vi "Get Hardware Version.vi"(0 "PCB":u32, 1 "Decode":u32, 2 "dummy1":u32, 3 "dummy2":u32, 4 "CameraFirmwareVersion":u32, 5 "CameraFirmwareBuild":u32, 7 "error in (no error)":errorcluster) -> (20 "PCB out":u32, 21 "Decode out":u32, 22 "dummy1 out":u32, 23 "dummy2 out":u32, 24 "CameraFirmwareVersion out":u32, 25 "CameraFirmwareBuild out":u32, 26 "function return":u32, 27 "error out":errorcluster)   [LabVIEW 2014, in "atmcd32d.lvlib"]
doc: "unsigned int WINAPI GetHardwareVersion(unsigned int * PCB, unsigned int * Decode, unsigned int * dummy1, unsigned int * dummy2, unsigned int * CameraFirmwareVersion, unsigned int * CameraFirmwareBuild);"
uses:
  atmcd32d.lvlib
  atmcd32d.dll
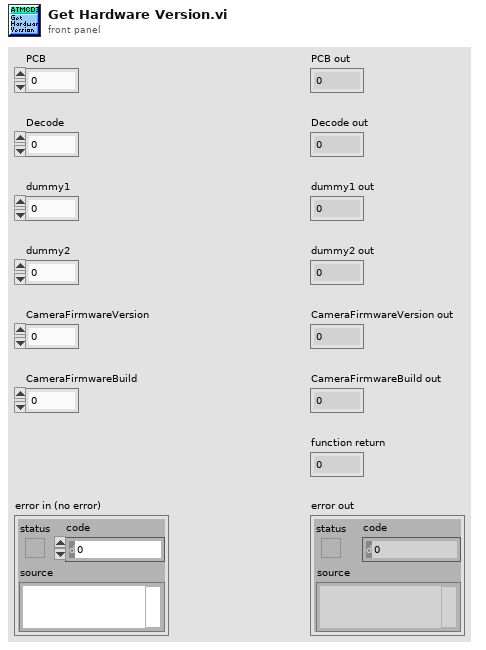
[diagram p1: front panel]
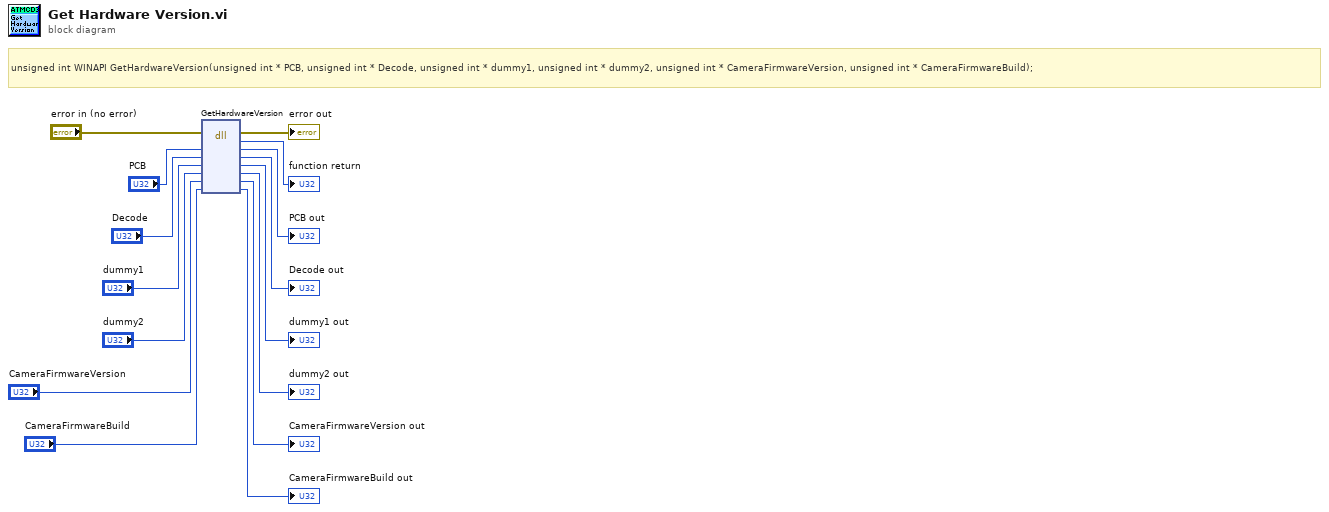
[diagram p0: block diagram]
diagram:
  # "unsigned int WINAPI GetHardwareVersion(unsigned int * PCB, unsigned int * Decode, unsigned int * dummy1, unsigned int * dummy2, unsigned int * CameraFirmwareVersion, unsigned int * CameraFirmwareBuild);"
  n1 = dll-call lib="C:/Users/Bakir/Documents/Lambda2-Testing/lib/Andorlib/atmcd32d.*" fn="GetHardwareVersion"(error in="error in (no error)", "PCB"="PCB", "Decode"="Decode", "dummy1"="dummy1", "dummy2"="dummy2", "CameraFirmwareVersion"="CameraFirmwareVersion", "CameraFirmwareBuild"="CameraFirmwareBuild") -> (error out=→"error out":errorcluster, →"function return":u32, "PCB"=→"PCB out":u32, "Decode"=→"Decode out":u32, "dummy1"=→"dummy1 out":u32, "dummy2"=→"dummy2 out":u32, "CameraFirmwareVersion"=→"CameraFirmwareVersion out":u32, "CameraFirmwareBuild"=→"CameraFirmwareBuild out":u32)  [unwired: 2 in, 1 out]
